vi "XboxInterface_Q.vi"() -> ()   [LabVIEW 2009]
uses:
  UDP Lib/UDP Network Location.ctl
  Remote Control/Motor Command.ctl
  Remote Control/Control Message.ctl
  Remote Control/Message Type.ctl
  <vilib>/Utility/inputDevices.llb/closeJoystick.vi
  <vilib>/Utility/inputDevices.llb/joystickAcquire.vi
panel:
  out "cRIO Down?":bool
  in  "stop":bool
  in  "Speed deadzone":i32=10240
  in  "Speed scaling factor":i32=250
  out "Comm Error":bool
  in  "Remote  Control/\nAutonomous":bool=TRUE
  in  "Controller Delta":dbl=256.0
  in  "Previous Values":cluster{"X axis":dbl, "Y axis rotation":dbl}
  in  "Turn scaling factor":i32=88
  in  "Turn deadzone":i32=10240
  out "Speed":i32(slide) scale=-128.0..128.0
  out "Turn":i32(slide) scale=-128.0..128.0
  out "joystick info":T1(array[cluster])=[{"axes total"=5, "buttons total"=10, "pov total"=1, "device name"="Controller (Xbox 360 Wireless Receiver for Windows)"}]
  out "axis info":T2={"X axis"=-5371, "Y axis"=-3971, "Z axis"=0, "X axis rotation"=-1504, "Y axis rotation"=-4411, "Z axis rotation"=0, "U axis"=0, "V axis"=0}
  out "direction info":T3={"pov 1"=-1, "pov 2"=-1, "pov 3"=-1, "pov 4"=-1}
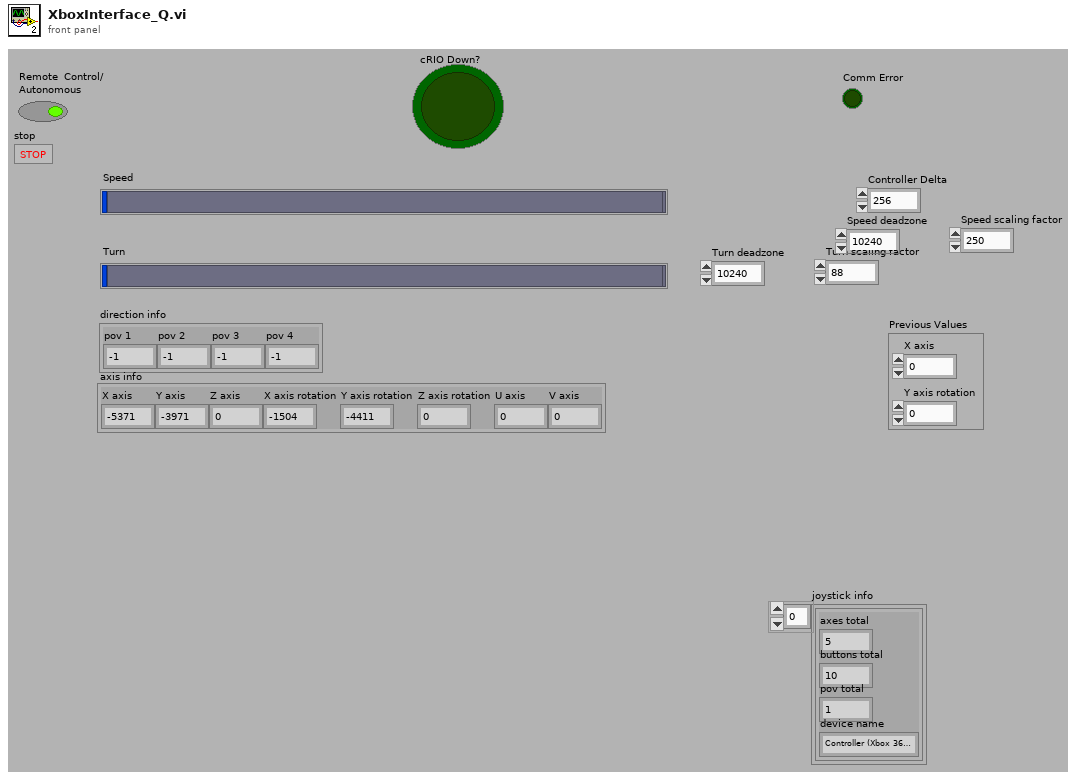
[diagram p1: front panel]
types:
  T1 = cluster{"axes total":u32, "buttons total":u32, "pov total":u32, "device name":string}[]
  T2 = cluster{"X axis":i32, "Y axis":i32, "Z axis":i32, "X axis rotation":i32, "Y axis rotation":i32, "Z axis rotation":i32, "U axis":i32, "V axis":i32}
  T3 = cluster{"pov 1":i32, "pov 2":i32, "pov 3":i32, "pov 4":i32}
  T4 = typedef "UDP Base.ctl" = cluster{"UDP Session":refnum<k16>, "UDP Socket Params":T5}
  T5 = typedef "UDP Socket Params.ctl" = cluster{"Local Port":u16, "Read Timeout":i32, "Write Timeout":i32}
  T6 = typedef "Message Type.ctl" = enum16{"Motor Command", "Debug Data"}
  T7 = typedef "Control Message.ctl" = cluster{"Motor Command":T8, "Time Stamp":timestamp, "Remote  Control/!Autonomous":bool, "Send Debug Data?":bool}
  T8 = typedef "Motor Command.ctl" = cluster{"Speed":i16, "Turn":i16}
  T9 = typedef "UDP Network Location.ctl" = cluster{"IP Address":string, "Port":u16}
  T10 = cluster{"button 1":bool, "button 2":bool, "button 3":bool, "button 4":bool, "button 5":bool, "button 6":bool, "button 7":bool, "button 8":bool, "button 9":bool, "button 10":bool, "button 11":bool, "button 12":bool, "button 13":bool, "button 14":bool, "button 15":bool, "button 16":bool, "button 17":bool, "button 18":bool, "button 19":bool, "button 20":bool, "button 21":bool, "button 22":bool, "button 23":bool, "button 24":bool, "button 25":bool, "button 26":bool, "button 27":bool, "button 28":bool, "button 29":bool, "button 30":bool, "button 31":bool, "button 32":bool}
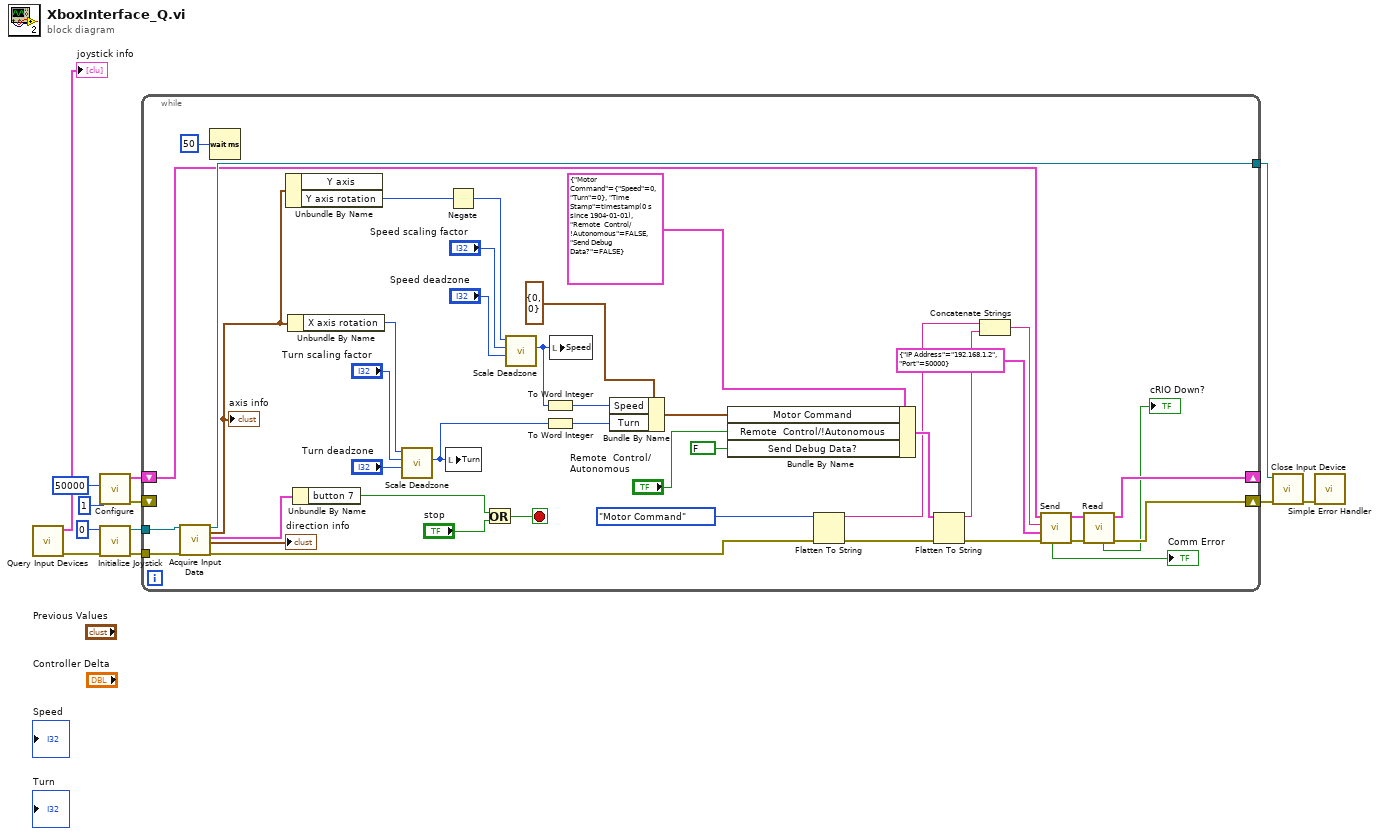
[diagram p0: block diagram]
diagram:
  n1 = call <vilib>:"Query Input Devices.vi"() -> ("error out"=w7:errorcluster, "joystick info"=→"joystick info":T1)  [unwired: 1 in, 9 out]
  n2 = call "Configure.vi"("Read Timeout"=1, "Local Port"=u16 50000) -> ("error out"=w4:errorcluster, "UDP Base out"=w3:T4)  [unwired: 8 in]
  n3 = call <vilib>:"Initialize Joystick.vi"("error in (no error)"=w7, "device index"=0) -> ("error out"=w10:errorcluster, "device ID"=w11:refnum<k1>)  [unwired: 8 out]
  n4 = while {
    tunnel: w11 -> [w54]
    tunnel: w10 -> [w53]
    tunnel: [w52] -> w9
    shift-right: [w14] -> _
    shift-left: w3 -> [w46]
    shift-right: [w15] -> w2
    shift-left: w4 -> [_]
    stop <- w19 stop-if-true
    n5 = call-poly <vilib>:"Acquire Input Data.vi"("device ID"=w54, "error in (no error)"=w53) -> ("device ID"=w52:refnum<k1>, "axis info"=w48:T2, "button info"=w51:T10, "direction info"=→"direction info":T3, "error out"=w29:errorcluster)  [unwired: 13 out]
    "axis info" <- w48
    n6 = Wait (ms)(milliseconds to wait=u32 50 ("millisecond multiple")) -> ()  [unwired: 1 out]
    n7 = Unbundle By Name(w48) -> ("Y axis rotation"=w44:i32)  [unwired: 1 out]
    n8 = Unbundle By Name(w48) -> ("X axis rotation"=w45:i32)
    n9 = Unbundle By Name(w51) -> ("button 7"=w20:bool)
    n10 = call "Scale Deadzone.vi"("deadzone"="Turn deadzone", "scaling factor"="Turn scaling factor", "input value"=w45) -> ("output value"=w22:i32)  [unwired: 8 in]
    n11 = local write "Turn"(w22) -> ()
    n12 = Negate(x=w44) -> (-x=w43:i32)
    n13 = Or(x=w20, y="stop") -> (x .or. y?=w19:bool)
    n14 = call "Scale Deadzone.vi"("deadzone"="Speed deadzone", "scaling factor"="Speed scaling factor", "input value"=w43) -> ("output value"=w41:i32)  [unwired: 8 in]
    n15 = To Word Integer(number=w41) -> (16bit integer=w21:i16)
    n16 = To Word Integer(number=w22) -> (16bit integer=w23:i16)
    n17 = local write "Speed"(w41) -> ()
    n18 = Bundle By Name(cluster=T8 {"Speed"=0, "Turn"=0} ("Motor Command"), "Speed"=w21, "Turn"=w23) -> (w39:T8)
    n19 = Bundle By Name(cluster=T7 {"Motor Command"={"Speed"=0, "Turn"=0}, "Time Stamp"=timestamp(0 s since 1904-01-01), "Remote  Control/!Autonomous"=FALSE, "Send Debug Data?"=FALSE} ("Control Cluster"), "Motor Command"=w39, "Remote  Control/!Autonomous"="Remote  Control/\nAutonomous", "Send Debug Data?"=FALSE ("Debug/Production")) -> (w36:T7)
    n20 = Flatten To String(anything=Message_Type."Motor Command" ("Message Type"), error in (no error)=w29) -> (data string=w25:string, error out=w28:errorcluster)  [unwired: 2 in, 1 out]
    n21 = Flatten To String(anything=w36, error in (no error)=w28) -> (data string=w24:string, error out=w30:errorcluster)  [unwired: 2 in, 1 out]
    n22 = Concatenate Strings(w25, w24) -> (w27:string)
    n23 = call "Send.vi"("error in (no error)"=w30, "Destination Location"=T9 {"IP Address"="192.168.1.2", "Port"=50000}, "Send Data"=w27, "UDP Base in"=w46) -> ("error out"=w16:errorcluster, "UDP Base out"=w17:T4, "Comm Error"=→"Comm Error":bool)  [unwired: 5 in]
    n24 = call "Read.vi"("error in (no error)"=w16, "UDP Base in"=w17) -> ("error out"=w15:errorcluster, "UDP Base out"=w14:T4, "Timeout"=→"cRIO Down?":bool)  [unwired: 4 in, 3 out]
  }
  n25 = call-poly <vilib>:"Close Input Device.vi"("error in (no error)"=w2, "device ID"=w9) -> ("error out"=w6:errorcluster)  [unwired: 8 out]
  n26 = call <vilib>:"Simple Error Handler.vi"("error in (no error)"=w6) -> ()  [unwired: 1 in, 8 out]
